vi "LABVIEW.vi"() -> ()   [LabVIEW 2017]
uses:
  <vilib>/picture/picture.llb/imagedata.ctl
  <vilib>/Instr/_visa.llb/VISA Configure Serial Port (Instr).vi
  <vilib>/addons/control/pid/pid.llb/PID (DBL).vi
  <vilib>/Utility/file.llb/Write To Spreadsheet File (DBL).vi
  <vilib>/addons/control/pid/NI_PID_pid.lvlib
panel:
  out "image data 2":T1
  out "image data":T1
  in  "?":enum32{"Configuração", "Análise", "Debug"}(tab)
  in  "Caminho \ndo Arquivo":path
  in  "PORTA COM":refnum<visa-resource-name>
  in  "PARÂMETROS PID":T2={"GANHO PROPORCIONAL (Kp)"=1.0, "TEMPO INTEGRAL (Ti, min)"=0.01, "TEMPO DERIVATIVO (Td, min)"=0.0} {"TEMPO DERIVATIVO (Td, min)" format="%.7f"; "TEMPO INTEGRAL (Ti, min)" format="%.2f"; "GANHO PROPORCIONAL (Kp)" format="%.3f"}
  in  "OUTPUT RANGE":cluster{"MÁX.":dbl, "MIN.":dbl}={"MÁX."=100.0, "MIN."=-100.0} {"MIN." format="%.2f"; "MÁX." format="%.2f"}
  in  "TEMPO (ms)":u32
  out "new picture 2":picture
  in  "IMAGEM DA ABA DE DEBUG":path
  in  "IMAGEM DA ABA CONFIGURA敲O":path
  out "RESPOSTA":dbl
  in  "GRAVAR":bool
  in  "SETPOINT":dbl(slide) scale=0.0..100.0
  in  "?":bool
  out "?":cluster{"SETPOINT":dbl, dbl}(graph)
  out "TEMPERATURA":dbl
  out "TEMPO (s)":dbl
  out "RESPOSTA":dbl(graph)
  out "PACOTE RECEBIDO":string
  out "PACOTE ENVIADO":string
  out "new picture":picture
  # "IMAGEM DA ABA CONFIGURA敲O"
  # "IMAGEM DA ABA DEBUG"
  # "SETPOINT"
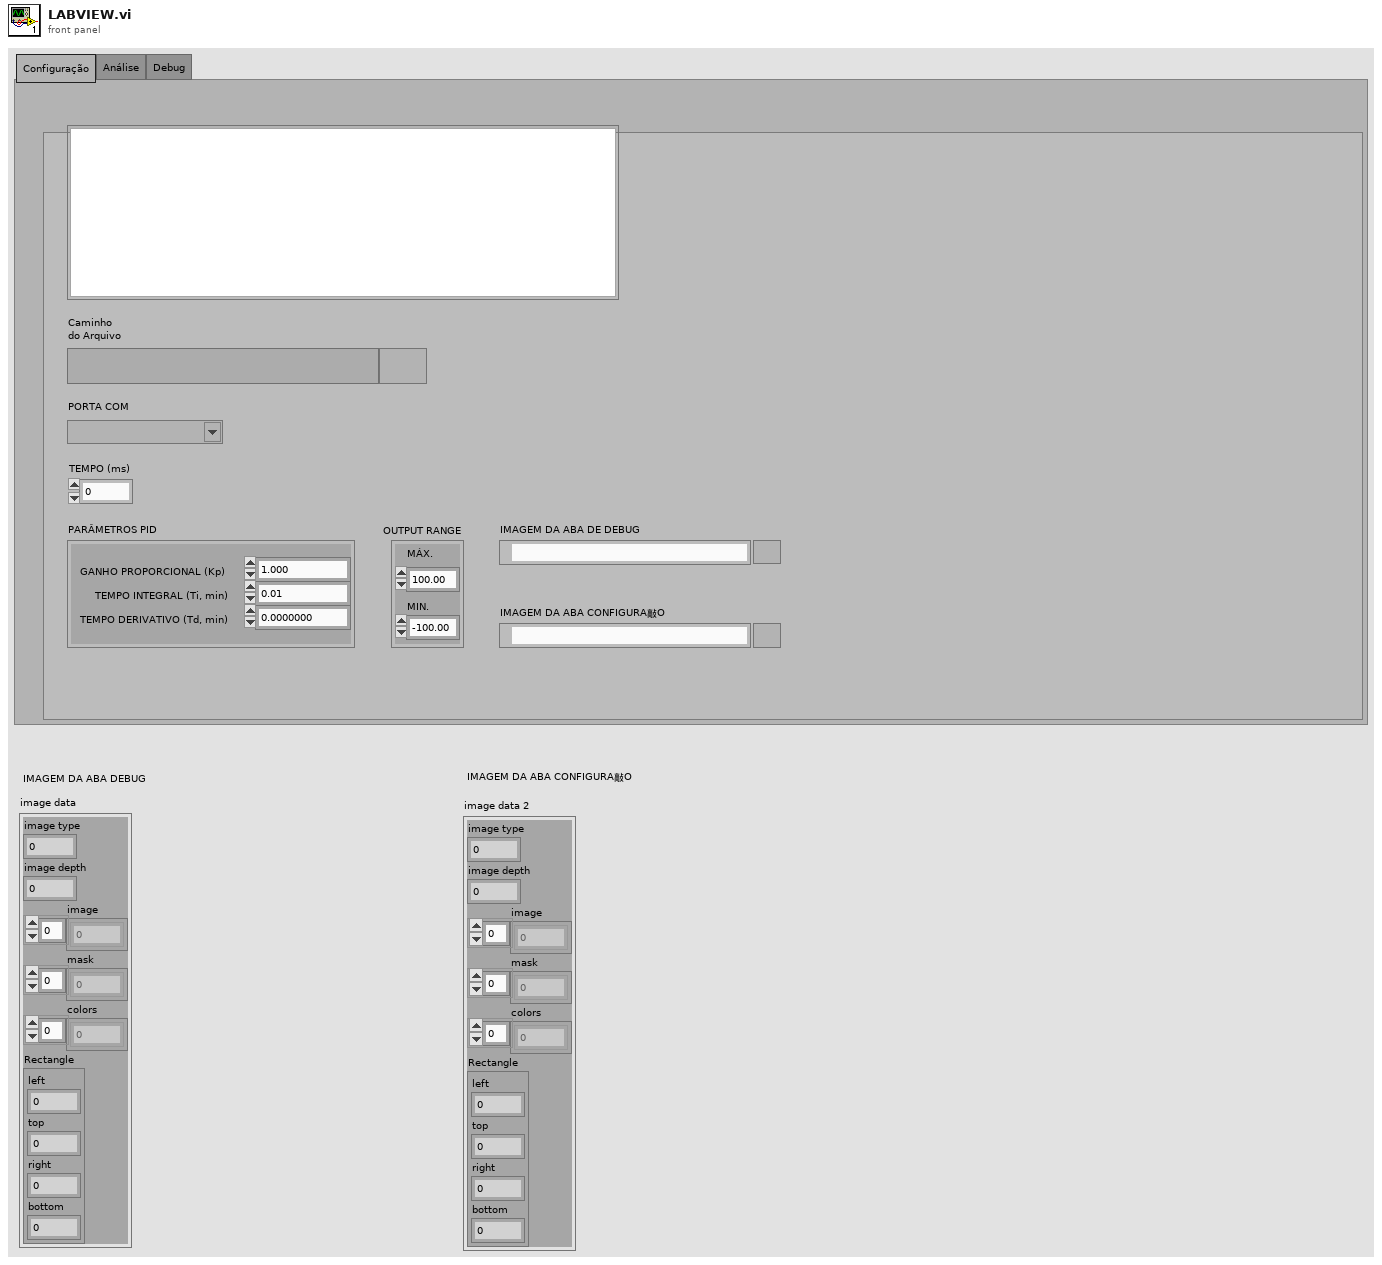
[diagram p1: front panel]
types:
  T1 = typedef "imagedata.ctl" = cluster{"image type":i32, "image depth":i32, "image":u8[], "mask":u8[], "colors":u32[], "Rectangle":cluster{"left":i16, "top":i16, "right":i16, "bottom":i16}}
  T2 = cluster{"GANHO PROPORCIONAL (Kp)":dbl, "TEMPO INTEGRAL (Ti, min)":dbl, "TEMPO DERIVATIVO (Td, min)":dbl}
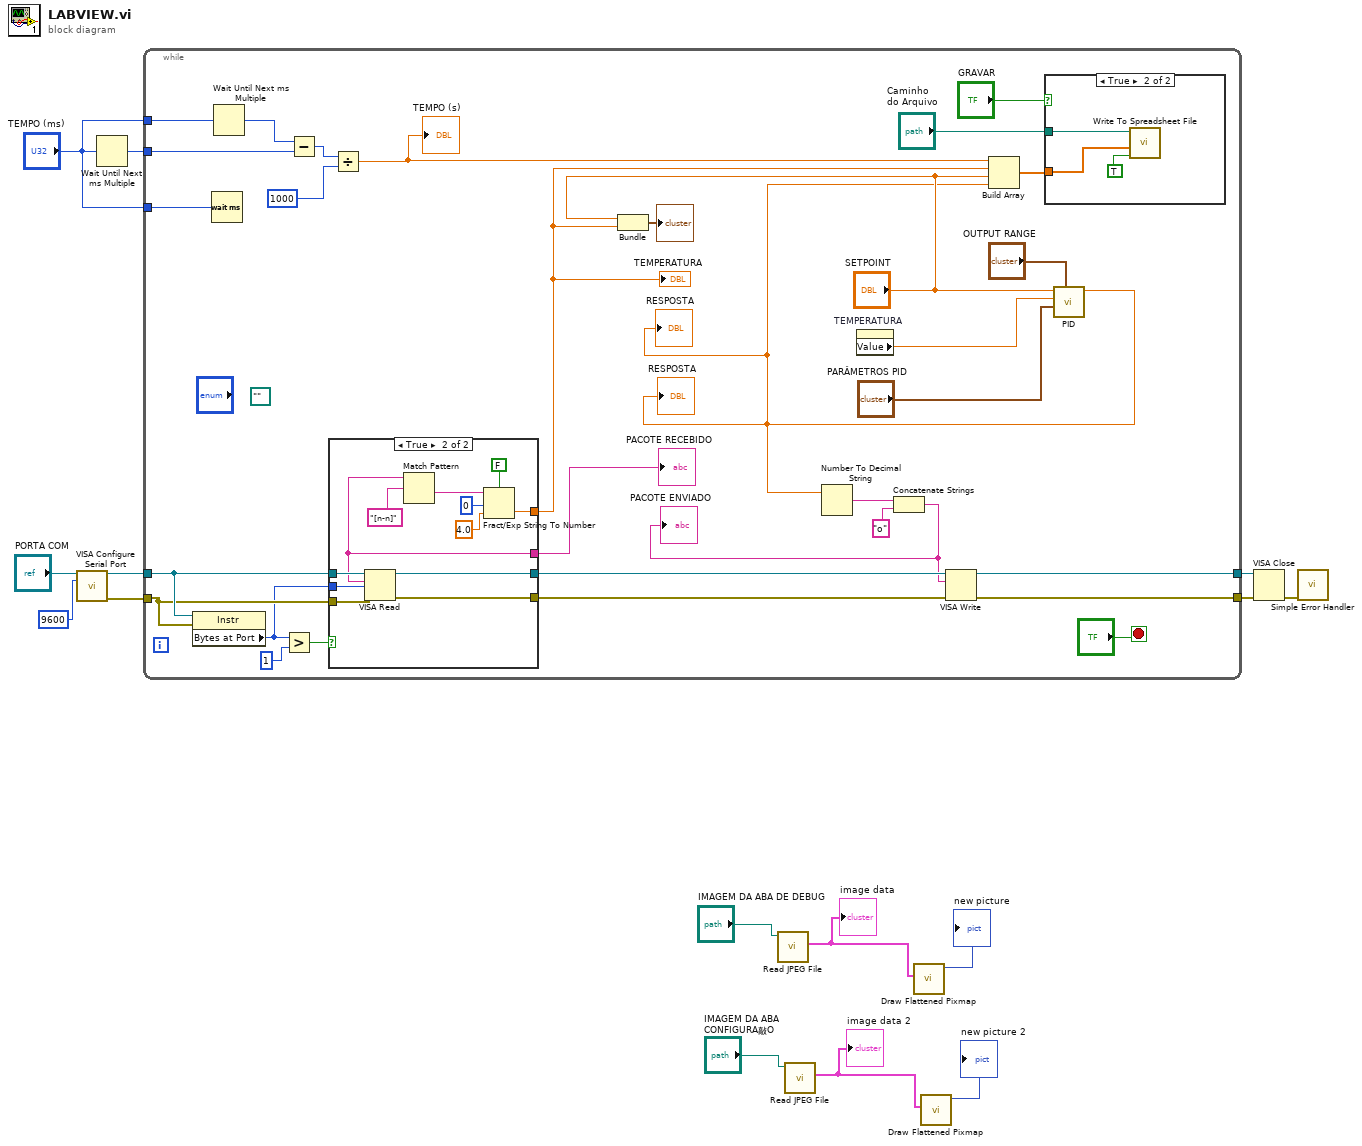
[diagram p0: block diagram]
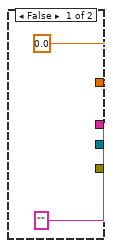
[diagram p3: hidden frame]
diagram:
  n1 = call-poly "VISA Configure Serial Port"("VISA resource name"="PORTA COM", "baud rate (9600)"=u32 9600) -> ("VISA resource name out"=w15:refnum<visa-resource-name>, "error out"=w14:errorcluster)  [unwired: 12 in]
  n2 = Wait Until Next ms Multiple(millisecond multiple="TEMPO (ms)") -> (millisecond timer value=w8:u32)
  n3 = while {
    tunnel: w15 -> [w44]
    tunnel: w14 -> [w43]
    tunnel: [w39] -> w10
    tunnel: [w38] -> w9
    tunnel: w8 -> [w30]
    tunnel: "TEMPO (ms)" -> [w20]
    tunnel: "TEMPO (ms)" -> [w19]
    stop <- "?" stop-if-true
    (unwired) path ""
    n4 = property class="Instr"(reference=w44, error in=w43) -> ("Bytes at Port"=w41:u32)  [unwired: 2 out]
    n5 = Wait (ms)(milliseconds to wait=w20) -> ()  [unwired: 1 out]
    n6 = Wait Until Next ms Multiple(millisecond multiple=w19) -> (millisecond timer value=w33:u32)
    n7 = Greater?(x=w41, y=u32 1) -> (0:w42:bool)
    n8 = Subtract(x=w33, y=w30) -> (x-y=w32:u32)
    n9 = case shown="True" w42 {
      tunnel: w44 -> [_ w63]
      tunnel: w43 -> [_ w62]
      tunnel: w41 -> [_ w61]
      tunnel: [_ w60] -> w40
      tunnel: [_ w59] -> w37
      tunnel: [0.0 w54] -> w18
      tunnel: ["" ("read buffer") w52] -> w16
      frame False {
      }
      frame True {
        n10 = VISA Read(VISA resource name=w63, byte count=w61, error in (no error)=w62) -> (VISA resource name out=w60:refnum<visa-resource-name>, read buffer=w52:string, error out=w59:errorcluster)  [unwired: 1 out]
        n11 = Match Pattern(string=w52, regular expression="[n-n]") -> (after substring=w53:string)  [unwired: 1 in, 3 out]
        n12 = Fract/Exp String To Number(use system decimal point (T)=FALSE, string=w53, offset=0, default (0 dbl)=4.0 ("default (0 DBL)")) -> (number=w54:dbl)  [unwired: 1 out]
      }
    }
    "TEMPERATURA" <- w18
    "PACOTE RECEBIDO" <- w16
    n13 = Divide(x=w32, y=u32 1000) -> (x/y=w26:dbl)
    "TEMPO (s)" <- w26
    n14 = Bundle("SETPOINT"="SETPOINT", w18) -> (→"?":cluster{"SETPOINT":dbl, dbl})  [unwired: 1 in]
    n15 = property on="TEMPERATURA" class="DigNum (strict)"() -> ("Value"=w23:dbl)  [unwired: 2 in, 2 out]
    n16 = call-poly <vilib>:"PID.vi"("output range"="OUTPUT RANGE", "PID gains"="PARÂMETROS PID", "process variable"=w23, "setpoint"="SETPOINT") -> ("output"=w17:dbl)  [unwired: 6 in, 1 out]
    "RESPOSTA" <- w17
    "RESPOSTA" <- w17
    n17 = Number To Decimal String(number=w17) -> (decimal integer string=w34:string)  [unwired: 1 in]
    n18 = Concatenate Strings(w34, "o" ("string")) -> (w35:string)
    "PACOTE ENVIADO" <- w35
    n19 = VISA Write(VISA resource name=w40, write buffer=w35, error in (no error)=w37) -> (VISA resource name out=w39:refnum<visa-resource-name>, error out=w38:errorcluster)  [unwired: 1 out]
    n20 = Build Array(w26, w18, "SETPOINT", w17) -> (w28:dbl[])
    n21 = case shown="True" "GRAVAR" {
      tunnel: "Caminho \ndo Arquivo" -> [_ w47]
      tunnel: w28 -> [_ w49]
      frame False {
      }
      frame True {
        n22 = call-poly <vilib>:"Write To Spreadsheet File.vi"("append to file? (new file:F)"=TRUE, "1D data"=w49, "file path (dialog if empty)"=w47) -> ()  [unwired: 5 in, 1 out]
      }
    }
  }
  n23 = call <vilib>:"Read JPEG File.vi"("path to JPEG file"="IMAGEM DA ABA DE DEBUG") -> ("image data"=w2:T1)  [unwired: 8 in, 2 out]
  "image data" <- w2
  n24 = call <vilib>:"Read JPEG File.vi"("path to JPEG file"="IMAGEM DA ABA CONFIGURA敲O") -> ("image data"=w5:T1)  [unwired: 8 in, 2 out]
  "image data 2" <- w5
  n25 = call <vilib>:"Draw Flattened Pixmap.vi"("image data"=w2) -> ("new picture"=→"new picture":picture)  [unwired: 8 in]
  n26 = call <vilib>:"Draw Flattened Pixmap.vi"("image data"=w5) -> ("new picture"=→"new picture 2":picture)  [unwired: 8 in]
  n27 = VISA Close(VISA resource name=w10, error in (no error)=w9) -> (error out=w11:errorcluster)
  n28 = call <vilib>:"Simple Error Handler.vi"("error in (no error)"=w11) -> ()  [unwired: 4 in, 5 out]
